vi "GetECLibDllPath.vi"(8 "error in (no error)":errorcluster, 11 "DLLPath":path) -> (0 "error out":errorcluster, 3 "ECLibDLLPath":path)   [LabVIEW 2022 SP3, in "EClib functions.lvlib"]
uses:
  EClib functions.lvlib
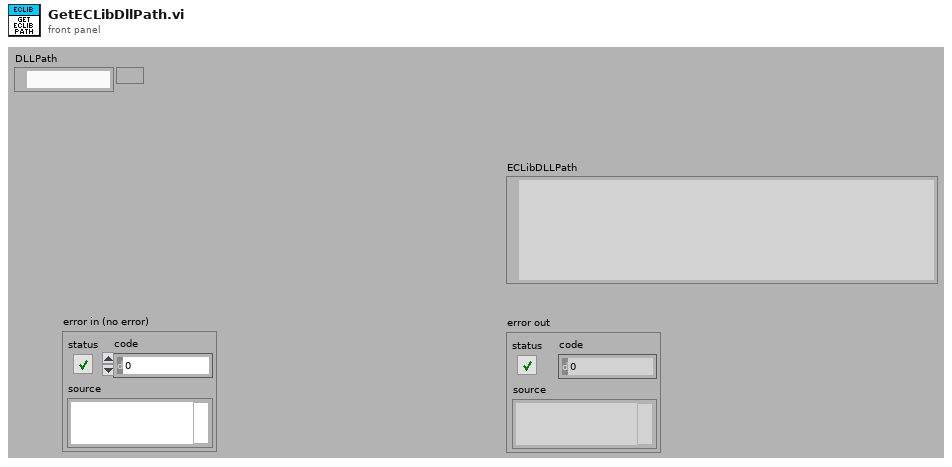
[diagram p1: front panel]
types:
  T1 = enum32{"invalid app kind", "Development System", "Run Time System", "Student Edition", "Embedded LabVIEW", "Evaluation", "Custom"}
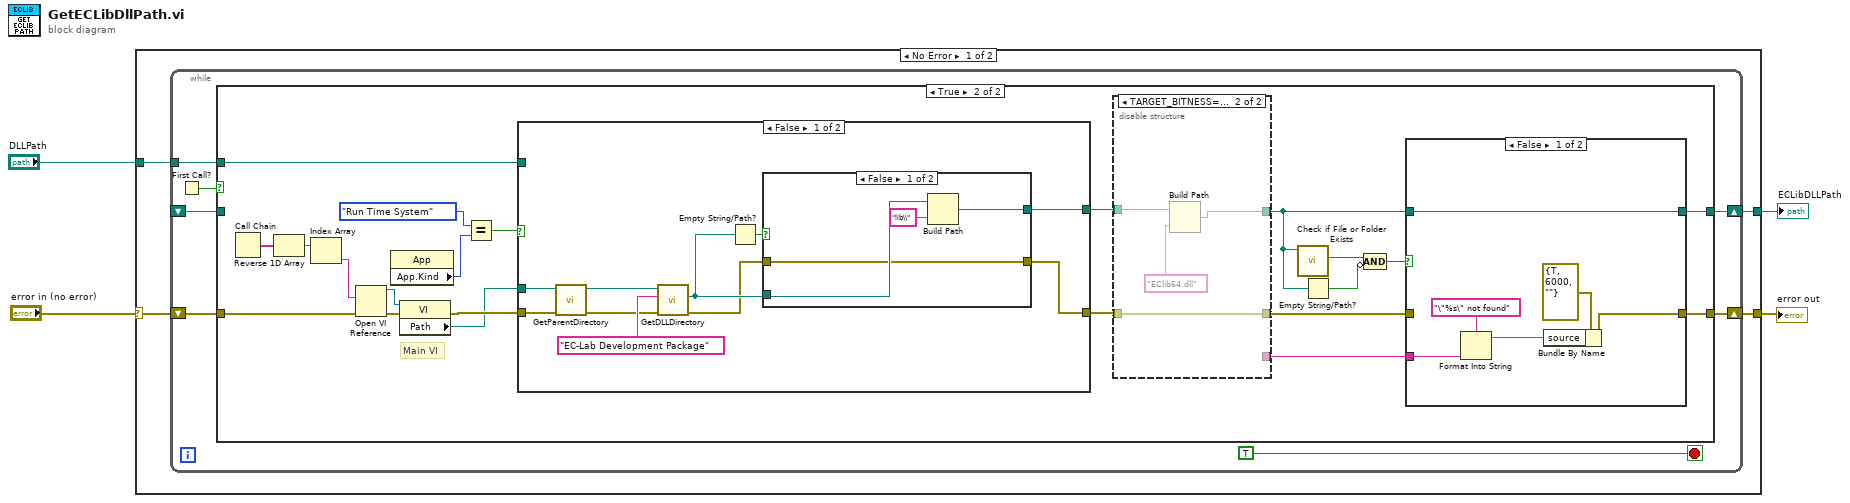
[diagram p0: block diagram]
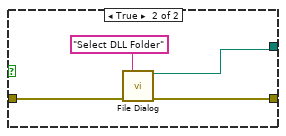
[diagram p3: hidden frame]
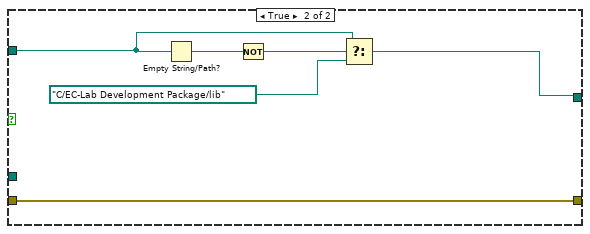
[diagram p4: hidden frame]
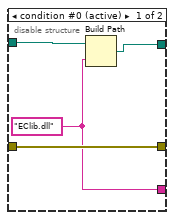
[diagram p6: hidden frame]
diagram:
  n1 = case shown="No Error" "error in (no error)" {
    selector: "error in (no error)" -> [w7 w80]
    tunnel: [w8 _] -> w4
    tunnel: [w6 w80] -> w2
    tunnel: "DLLPath" -> [w5 _]
    frame No Error {
      n2 = while {
        shift-right: [w13] -> w6
        shift-left: w7 -> [w14]
        shift-right: [w15] -> w8
        shift-left: _ -> [w10]
        tunnel: w5 -> [w9]
        stop <- TRUE stop-if-true
        n3 = First Call?() -> (First Call?: T/F=w11:bool)
        n4 = case shown="True" w11 {
          tunnel: [w17 w27] -> w15
          tunnel: w14 -> [w16 w34]
          tunnel: [w16 w30] -> w13
          tunnel: w10 -> [w17 _]
          tunnel: w9 -> [_ w18]
          frame False {
          }
          frame True {
            # "Main VI"
            n5 = Call Chain() -> (call chain=w36:string[])
            n6 = Reverse 1D Array(array=w36) -> (reversed array=w35:string[])
            n7 = Index Array(array=w35) -> (element=w37:string)  [unwired: 1 in]
            n8 = Open VI Reference(vi path=w37, error in (no error)=w34) -> (vi reference=w39:refnum<vi>, error out=w38:errorcluster)  [unwired: 4 out]
            n9 = property class="App"() -> ("App.Kind"=w24:T1)  [unwired: 2 in, 2 out]
            n10 = property class="VI"(reference=w39, error in=w38) -> (error out=w20:errorcluster, "Path"=w19:path)  [unwired: 1 out]
            n11 = Equal?(x=T1."Run Time System" ("Application:Kind"), y=w24) -> (x = y?=w23:bool)
            n12 = case shown="False" w23 {
              tunnel: [w40 w63] -> w22
              tunnel: [w44 w59] -> w21
              tunnel: w20 -> [w48 w63]
              tunnel: w19 -> [w47 _]
              tunnel: w18 -> [_ w60]
              frame False {
                n13 = call "GetParentDirectory.vi"("error in"=w48, "VIPath"=w47) -> ("error out"=w46:errorcluster, "VIRelativePath"=w45:path)  [unwired: 7 in, 1 out]
                n14 = call "GetDLLDirectory.vi"("error in (no error)"=w46, "DLLDirectoryName"="EC-Lab Development Package", "AppParentDirectory"=w45) -> ("error out"=w41:errorcluster, "DLLDirectory"=w43:path)  [unwired: 6 in, 1 out]
                n15 = Empty String/Path?(string/path=w43) -> (empty?=w42:bool)
                n16 = case shown="False" w42 {
                  tunnel: [w52 w56] -> w44
                  tunnel: w43 -> [w51 _]
                  tunnel: w41 -> [w50 w55]
                  tunnel: [w50 w54] -> w40
                  frame False {
                    n17 = Build Path(base path=w51, name or relative path="lib\\") -> (appended path=w52:path)
                  }
                  frame True {
                    n18 = call "File Dialog"("prompt"="Select DLL Folder", "error in"=w55) -> ("selected path"=w56:path, "error out"=w54:errorcluster)  [unwired: 10 in, 2 out]
                  }
                }
              }
              frame True {
                n19 = Empty String/Path?(string/path=w60) -> (empty?=w62:bool)
                n20 = Not(x=w62) -> (.not. x?=w61:bool)
                n21 = Select(t=w60, s=w61, f=path "C:/EC-Lab Development Package/lib" ("base path")) -> (s? t:f=w59:path)
              }
            }
            n22 = disable-structure shown="TARGET_BITNESS==64" {
              disable-tunnel: [w75 w79] -> w28
              disable-tunnel: w22 -> [w74 w78]
              disable-tunnel: [w74 w78] -> w31
              disable-tunnel: w21 -> [w72 w76]
              disable-tunnel: [w73 _] -> w26
              frame condition #0 (active) {
                w73 = "EClib.dll" ("name or relative path")
                n23 = Build Path(base path=w72, name or relative path=w73) -> (appended path=w75:path)
              }
              frame condition #1 {
                n24 = Build Path(base path=w76, name or relative path="EClib64.dll") -> (appended path=w79:path)
              }
            }
            n25 = call <vilib>:"Check if File or Folder Exists.vi"("path"=w28) -> ("file or folder exists?"=w33:bool)  [unwired: 8 in, 2 out]
            n26 = Empty String/Path?(string/path=w28) -> (empty?=w32:bool)
            n27 = Compound Arithmetic op=AND(w33, invert w32) -> (w29:bool)
            n28 = case shown="False" w29 {
              tunnel: w31 -> [_ w71]
              tunnel: [w67 w71] -> w30
              tunnel: w28 -> [w69 w70]
              tunnel: [w69 w70] -> w27
              tunnel: w26 -> [w66 _]
              frame False {
                n29 = Format Into String(format string="\"%s\" not found", w66) -> (resulting string=w64:string)  [unwired: 2 in, 1 out]
                n30 = Bundle By Name(cluster=errorcluster {"status"=TRUE, "code"=6000, "source"=""} ("error out"), "source"=w64) -> (w67:errorcluster)
              }
              frame True {
              }
            }
          }
        }
      }
    }
    frame Error {
    }
  }
  "ECLibDLLPath" <- w4
  "error out" <- w2
